vi "读配置文件全局.vi"() -> ()   [LabVIEW 2013]
panel:
  in  "选项卡控件":enum32{"主板", "从板"}(tab)
  out "从板个数判定":bool
  out "电池充放电次数判定":bool
  out "充放电安时判定":bool
  out "电池包组号判定":bool
  out "电池信息1判定":bool
  out "充电控制参数判定":bool
  out "加热控制参数判定":bool
  out "三级故障判定":bool
  out "二级故障判定":bool
  out "一级故障判定":bool
  out "SOH判定":bool
  out "车牌号判定":bool
  out "配置文件版本判定":bool
  out "电池额定实际容量判定":bool
  out "SOC判定":bool
  out "保险位置判定":bool
  out "温度起始值判定":bool
  out "温度个数判定":bool
  out "电压起始值判定":bool
  out "通道电压数判定":bool
  out "电压个数判定":bool
  out "产品编号判定":bool
  in  "电池信息":T1={"电池串联"=0.0, "电池并联"=0.0, "累计放电总安时"=0.0, "电池包额定容量"=0.0, "电池包额定能量"=0.0, "电池包额定总电压"=0.0, "累计充电总安时"=0.0, "电池充满次数"=0.0, "电池放空次数"=0.0, "电池充电次数"=0.0, "电池生产日期"="", "电池厂家"="", "电池类型"="", "电池包组号"="", "电池包产权标识"="122", "电池应用车型"="123", "实际容量"=0.0}
  out "充电控制参数":dbl[](array[numeric])
  out "加热控制参数":dbl[](array[numeric])
  out "三级故障":sgl[](array[numeric])
  out "二级故障":sgl[](array[numeric])
  out "一级故障":sgl[](array[numeric])
  in  "项目信息":T2
  out "从板个数":dbl
  out "表格输入":string[](array[string])
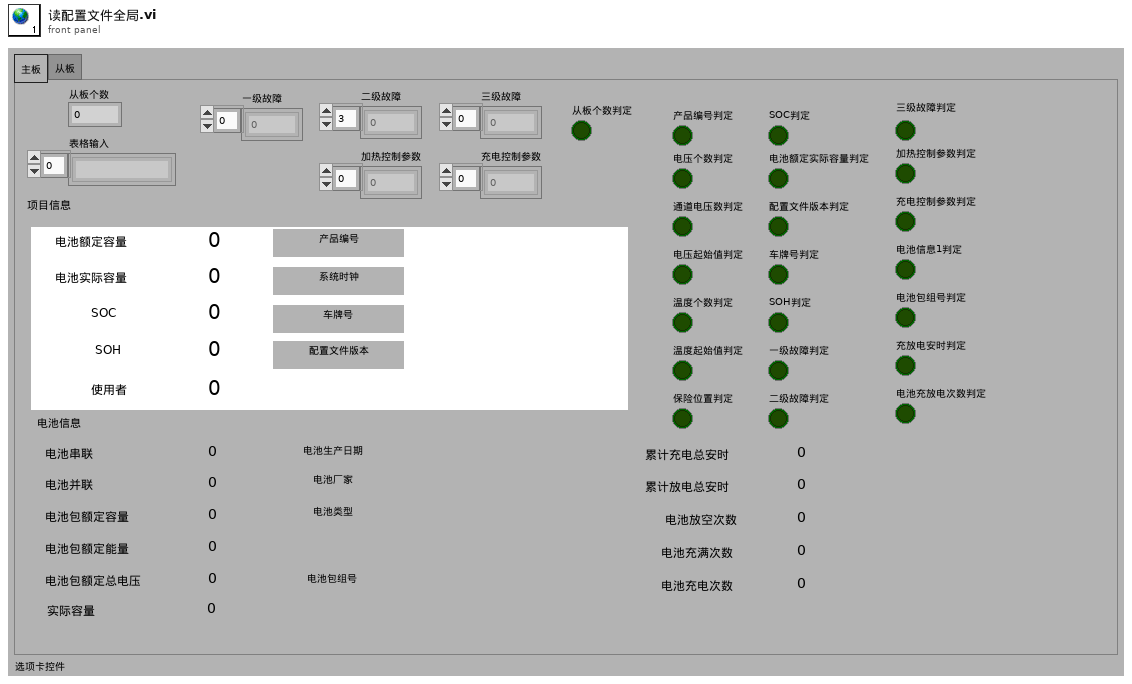
[diagram p1: front panel]
types:
  T1 = cluster{"电池串联":dbl, "电池并联":dbl, "累计放电总安时":dbl, "电池包额定容量":dbl, "电池包额定能量":dbl, "电池包额定总电压":dbl, "累计充电总安时":dbl, "电池充满次数":dbl, "电池放空次数":dbl, "电池充电次数":dbl, "电池生产日期":string, "电池厂家":string, "电池类型":string, "电池包组号":string, "电池包产权标识":string, "电池应用车型":string, "实际容量":dbl}
  T2 = cluster{"电池额定容量":dbl, "使用者":dbl, "电池实际容量":dbl, "车牌号":string, "配置文件版本":string, "SOH":dbl, "SOC":dbl, "产品编号":string, "系统时钟":string}
diagram:
